vi "Add Block Diagram Content.vi"(8 "error in (no error)":errorcluster, 10 "ModuleLoop":T1, 11 "EST Output in":refnum<class "EST Output.lvclass">) -> (0 "error out":errorcluster, 2 "Term Refnum":refnum<vi>, 3 "EST Output out":refnum<class "EST Output.lvclass">)   [LabVIEW 2015, in "EST Output.lvclass"]
uses:
  EST Output.lvclass
  VI/VI/Module.Refs.ctl
  <vilib>/Utility/miscctls.llb/LVPointTypeDef.ctl
  EST Output.lvclass/EST Output.ctl
  Signal/Read IP Core Path.vi
  Signal/Read Signal Name.vi
  VI/Structures/Structures.lvclass
  VI/VI/VI.lvclass
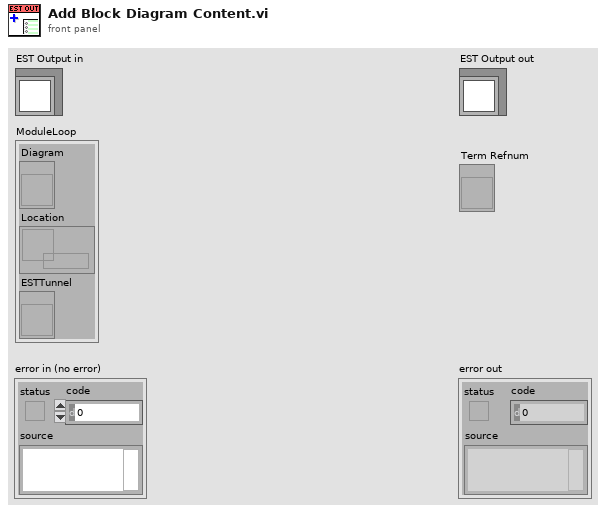
[diagram p1: front panel]
types:
  T1 = typedef "VI.lvclass/Module.Refs.ctl" = cluster{"Diagram":refnum<vi>, "Location":refnum<data-value>, "ESTTunnel":refnum<vi>}
  T2 = typedef "LVPointTypeDef.ctl" = cluster{"Horizontal":i16, "Vertical":i16}
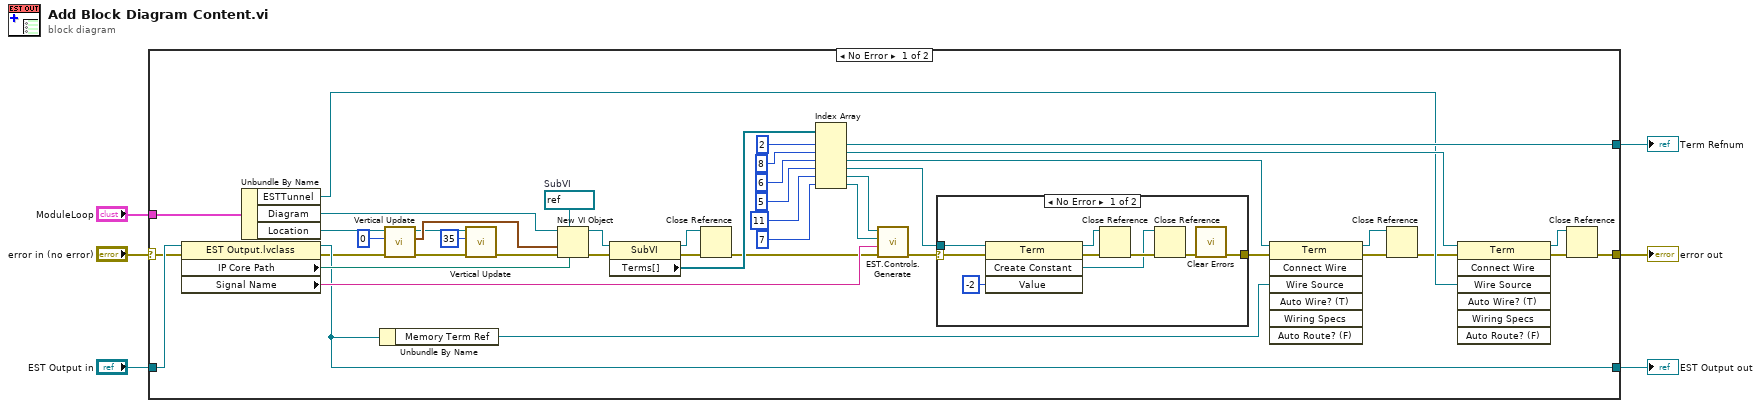
[diagram p0: block diagram]
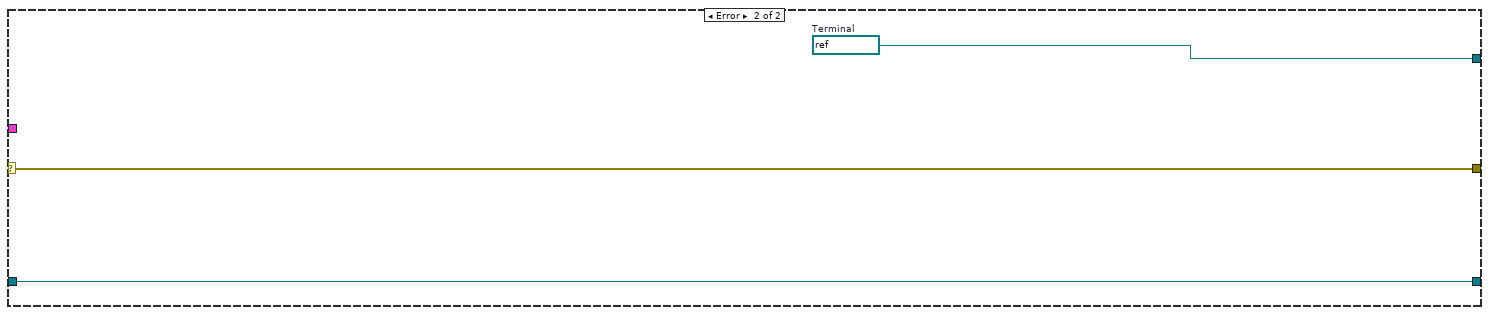
[diagram p3: hidden frame]
diagram:
  n1 = case shown="No Error" "error in (no error)" {
    selector: "error in (no error)" -> [w16 w63]
    tunnel: "ModuleLoop" -> [w50 _]
    tunnel: [w10 w63] -> w5
    tunnel: [w32 w61] -> w4
    tunnel: "EST Output in" -> [w28 w62]
    tunnel: [w27 w62] -> w2
    frame No Error {
      w45 = refnum<vi> refnum  # SubVI
      n2 = property class="EST Output.lvclass"(reference=w28, error in=w16) -> (reference out=w27:refnum<class "EST Output.lvclass">, error out=w23:errorcluster, "IP Core Path"=w30:path, "Signal Name"=w31:string)
      n3 = Unbundle By Name(w50) -> ("ESTTunnel"=w17:refnum<vi>, "Diagram"=w18:refnum<vi>, "Location"=w25:refnum<data-value>)
      n4 = Unbundle By Name(w27) -> ("Memory Term Ref"=w29:refnum<vi>)
      n5 = call "Vertical Update.vi"("error in (no error)"=w23, "Vertical Change"=i16 0, "Location"=w25) -> ("error out"=w20:errorcluster, "location out"=w24:T2, "Location"=w21:refnum<data-value>)  [unwired: 6 in]
      n6 = call "Vertical Update.vi"("error in (no error)"=w20, "Vertical Change"=i16 35, "Location"=w21) -> ("error out"=w19:errorcluster)  [unwired: 6 in, 2 out]
      n7 = New VI Object(vi object class=w45, owner refnum=w18, position/next to=w24, 6:w30, 8:w19) -> (object refnum=w48:refnum<vi>, 0:w49:errorcluster)  [unwired: 3 in]
      n8 = property class="SubVI"(reference=w48, error in=w49) -> (reference out=w15:refnum<vi>, error out=w14:errorcluster, "Terms[]"=w46:refnum<vi>[])
      n9 = Close Reference(reference=w15, error in (no error)=w14) -> (error out=w13:errorcluster)
      n10 = Index Array(array=w46, index #1=2 ("index"), index #2=8 ("index"), index #3=6 ("index"), index #4=5 ("index"), index #5=11 ("index"), index #6=7 ("index")) -> (element #1=w32:refnum<vi>, element #2=w36:refnum<vi>, element #3=w39:refnum<vi>, element #4=w41:refnum<vi>, element #5=w34:refnum<vi>, element #6=w35:refnum<vi>)
      n11 = call "EST.Controls.Generate.vi"("error in (no error)"=w13, "IO Name"=w31, "Input.Ref"=w35, "Settings.Ref"=w34) -> ("error out"=w33:errorcluster)  [unwired: 7 in]
      n12 = case shown="No Error" w33 {
        selector: w33 -> [w57 w60]
        tunnel: w41 -> [w59 _]
        tunnel: [w54 w60] -> w40
        frame No Error {
          n13 = invoke class="Term" method="Create Constant"(reference=w59, error in=w57, "Value"=i8 -2 ("shift")) -> (reference out=w55:refnum<vi>, error out=w56:errorcluster, "Create Constant"=w51:refnum<vi>)  [unwired: 1 in, 1 out]
          n14 = Close Reference(reference=w55, error in (no error)=w56) -> (error out=w53:errorcluster)
          n15 = Close Reference(reference=w51, error in (no error)=w53) -> (error out=w52:errorcluster)
          n16 = call <vilib>:"Clear Errors.vi"("error in (no error)"=w52) -> ("error out"=w54:errorcluster)  [unwired: 5 in, 1 out]
        }
        frame Error {
        }
      }
      n17 = invoke class="Term" method="Connect Wire"(reference=w39, error in=w40, "Wire Source"=w29) -> (reference out=w9:refnum<vi>, error out=w8:errorcluster)  [unwired: 4 in, 5 out]
      n18 = Close Reference(reference=w9, error in (no error)=w8) -> (error out=w7:errorcluster)
      n19 = invoke class="Term" method="Connect Wire"(reference=w36, error in=w7, "Wire Source"=w17) -> (reference out=w12:refnum<vi>, error out=w11:errorcluster)  [unwired: 4 in, 5 out]
      n20 = Close Reference(reference=w12, error in (no error)=w11) -> (error out=w10:errorcluster)
    }
    frame Error {
      w61 = refnum<vi> refnum  # Terminal
    }
  }
  "error out" <- w5
  "EST Output out" <- w2
  "Term Refnum" <- w4
